vi "Version_2.0_Single_Column_Code.vi"() -> ()   [LabVIEW 2020] (continued)
                              frame #4 {
                                n4126 = while {
                                stop <- w4536 stop-if-true
                                n4127 = local read "Stopper that ends \nthe main loops"() -> (w4537:bool)
                                n4128 = local read "VISA Refnum in\nfor Pump"() -> (w4538:refnum<visa-resource-name>)
                                n4129 = case shown="True" w4537 {
                                frame False {
                                }
                                frame True {
                                n4130 = local read "VISA Refnum in\nfor Pump"() -> (w4539:refnum<visa-resource-name>)
                                n4131 = call "HardStopCurrentProcess (SubVI).vi"("VISA Refnum in"=w4539) -> ()  [unwired: 11 in]
                                }
                                }
                                n4132 = call "ProcessCompletionWaiterWithOutPut (SubVI).vi"("VISA Refnum in"=w4538) -> ("Boolean"=w4536:bool)  [unwired: 10 in]
                                }
                              }
                              frame #5 {
                                n4133 = local read "Buffer-B Dispense\nFlow Rate for Elution \ntubing pre-wash"() -> (w4543:dbl)
                                n4134 = local read "Buffer-B Pumping\nResolution"() -> (w4542:T2)
                                n4135 = local read "VISA Refnum in\nfor Pump"() -> (w4545:refnum<visa-resource-name>)
                                n4136 = local write "Pause Data Collection"(TRUE ("Pause Data Collection")) -> ()
                                n4137 = local read "Volume of Syringe"() -> (w4544:dbl)
                                n4138 = call "GoToAbsolutePosition(SubVI).vi"("Absolute Volume Position in Syringe (in ul)"=0.0 ("Volume to be Dispensed"), "Volume of Syringe"=w4544, "Resolution of Pumping"=w4542, "Flow Rate (ul/min)"=w4543, "VISA Refnum in"=w4545) -> ()  [unwired: 6 in, 1 out]
                              }
                              frame #6 {
                                n4139 = local read "VISA Refnum in\nfor Pump"() -> (w4549:refnum<visa-resource-name>)
                                n4140 = local read "Initial Plunger Position"() -> (w4548:dbl)
                                n4141 = local read "Volume of Syringe"() -> (w4546:dbl)
                                n4142 = local read "Buffer-B Pumping\nResolution"() -> (w4547:T2)
                                n4143 = while {
                                tunnel: w4548 -> [w4556]
                                tunnel: w4549 -> [w4555]
                                tunnel: w4547 -> [w4554]
                                tunnel: w4546 -> [w4553]
                                stop <- w4551 stop-if-true
                                n4144 = stacked-sequence {
                                tunnel: w4556 -> [w4563 _]
                                tunnel: w4555 -> [w4562 w4583]
                                tunnel: w4554 -> [w4561 _]
                                tunnel: w4553 -> [w4560 _]
                                tunnel: [_ w4581] -> w4551
                                frame #0 {
                                n4145 = call "AbsolutePlungerPosition (SubVI).vi"("VISA Refnum in"=w4562) -> ("Plunger Position"=w4559:i32)  [unwired: 10 in]
                                n4146 = case shown="\"Standard Pumping\", Default" w4561 {
                                tunnel: w4563 -> [w4568 w4577]
                                tunnel: w4559 -> [w4569 w4576]
                                tunnel: [w4567 w4574] -> w4558
                                tunnel: w4560 -> [w4566 w4575]
                                frame "Standard Pumping", Default {
                                n4147 = Subtract(x=w4568, y=w4569) -> (x-y=w4565:dbl)
                                n4148 = Absolute Value(x=w4565) -> (abs(x)=w4564:dbl)
                                n4149 = Multiply(x=w4564, y=w4566) -> (x*y=w4571:dbl)
                                n4150 = Divide(x=w4571, y=3000.0) -> (x/y=w4567:dbl)
                                }
                                frame "High Resolution Pumping" {
                                n4151 = Subtract(x=w4577, y=w4576) -> (x-y=w4573:dbl)
                                n4152 = Absolute Value(x=w4573) -> (abs(x)=w4572:dbl)
                                n4153 = Multiply(x=w4572, y=w4575) -> (x*y=w4579:dbl)
                                n4154 = Divide(x=w4579, y=24000.0) -> (x/y=w4574:dbl)
                                }
                                }
                                n4155 = local write "Volume being Injected \nin this process"(w4558) -> ()
                                }
                                frame #1 {
                                n4156 = call "LSPOneStatus (SubVI).vi"("VISA Refnum in"=w4583) -> ("read buffer"=w4585:string)  [unwired: 10 in]
                                n4157 = call <vilib>:"Trim Whitespace.vi"("string"=w4585) -> ("trimmed string"=w4584:string)  [unwired: 1 in]
                                n4158 = local read "Stopper that ends \nthe main loops"() -> (w4580:bool)
                                n4159 = Equal?(x=w4584, y="/0`\u0003") -> (x = y?=w4582:bool)
                                n4160 = Or(x=w4582, y=w4580) -> (x .or. y?=w4581:bool)
                                }
                                }
                                n4161 = Wait (ms)(milliseconds to wait=u32 100) -> ()  [unwired: 1 out]
                                n4162 = local read "Stopper that ends \nthe main loops"() -> (w4550:bool)
                                n4163 = case shown="True" w4550 {
                                frame False {
                                }
                                frame True {
                                n4164 = local read "VISA Refnum in\nfor Pump"() -> (w4557:refnum<visa-resource-name>)
                                n4165 = call "HardStopCurrentProcess (SubVI).vi"("VISA Refnum in"=w4557) -> ()  [unwired: 11 in]
                                }
                                }
                                }
                              }
                              frame #7 {
                                # "Change the pump port to Buffer-A1 for equilibriation of column-1"
                                n4166 = local read "VISA Refnum in\nfor Pump"() -> (w4588:refnum<visa-resource-name>)
                                n4167 = local read "Port for \nA1-Equilibriation"() -> (w4587:string)
                                n4168 = local write "Pause Data Collection"(TRUE ("Pause Data Collection")) -> ()
                                n4169 = Wait (ms)(milliseconds to wait=u32 500) -> ()  [unwired: 1 out]
                                n4170 = call "PortChanger (SubVI).vi"("Port Number"=w4587, "VISA Refnum in"=w4588) -> ()  [unwired: 10 in]
                              }
                              frame #8 {
                                n4171 = local read "VISA Refnum in\nfor Pump"() -> (w4592:refnum<visa-resource-name>)
                                n4172 = local write "Volume being Injected \nin this process"(0.0 ("Volume being Injected \nin this process")) -> ()
                                n4173 = call "ProcessCompletionWaiter (SubVI).vi"("VISA Refnum in"=w4592) -> ()  [unwired: 11 in]
                                n4174 = local write "Start the Process"(FALSE ("Start the Process")) -> ()
                              }
                            }
                          }
                          frame #7 {
                            # "Clean the tubing with Buffer-A1"
                            n4175 = local read "N-A1"() -> (w4594:i32)
                            n4176 = for {
                              N: w4594 -> [_]
                              n4177 = stacked-sequence {
                                frame #0 {
                                n4178 = local read "VISA Refnum in\nfor Pump"() -> (w4597:refnum<visa-resource-name>)
                                n4179 = local read "Port for \nA1-Equilibriation"() -> (w4596:string)
                                n4180 = call "PortChanger (SubVI).vi"("Port Number"=w4596, "VISA Refnum in"=w4597) -> ()  [unwired: 10 in]
                                }
                                frame #1 {
                                n4181 = local read "VISA Refnum in\nfor Pump"() -> (w4598:refnum<visa-resource-name>)
                                n4182 = call "ProcessCompletionWaiter (SubVI).vi"("VISA Refnum in"=w4598) -> ()  [unwired: 11 in]
                                }
                                frame #2 {
                                n4183 = local read "VISA Refnum in\nfor Pump"() -> (w4603:refnum<visa-resource-name>)
                                n4184 = local read "Apparent Volume\nof Syringe"() -> (w4599:dbl)
                                n4185 = local read "Volume of Syringe"() -> (w4600:dbl)
                                n4186 = call "RPickUp(SubVI).vi"("Volume to be picked up"=w4599, "Volume of Syringe"=w4600, "Resolution of PickUP"=T2."Standard Pumping", "PickUp Flow Rate (ul/min)"=150.0, "VISA Refnum in"=w4603) -> ()  [unwired: 6 in, 1 out]
                                }
                                frame #3 {
                                n4187 = local read "Stopper that ends \nthe main loops"() -> (w4604:bool)
                                n4188 = local read "VISA Refnum in\nfor Pump"() -> (w4605:refnum<visa-resource-name>)
                                n4189 = case shown="True" w4604 {
                                frame False {
                                }
                                frame True {
                                n4190 = local read "VISA Refnum in\nfor Pump"() -> (w4606:refnum<visa-resource-name>)
                                n4191 = call "HardStopCurrentProcess (SubVI).vi"("VISA Refnum in"=w4606) -> ()  [unwired: 11 in]
                                }
                                }
                                n4192 = call "ProcessCompletionWaiter (SubVI).vi"("VISA Refnum in"=w4605) -> ()  [unwired: 11 in]
                                }
                                frame #4 {
                                n4193 = local read "VISA Refnum in\nfor Pump"() -> (w4608:refnum<visa-resource-name>)
                                n4194 = call "PortChanger (SubVI).vi"("Port Number"="1", "VISA Refnum in"=w4608) -> ()  [unwired: 10 in]
                                }
                                frame #5 {
                                n4195 = local read "Stopper that ends \nthe main loops"() -> (w4609:bool)
                                n4196 = local read "VISA Refnum in\nfor Pump"() -> (w4610:refnum<visa-resource-name>)
                                n4197 = case shown="True" w4609 {
                                frame False {
                                }
                                frame True {
                                n4198 = local read "VISA Refnum in\nfor Pump"() -> (w4611:refnum<visa-resource-name>)
                                n4199 = call "HardStopCurrentProcess (SubVI).vi"("VISA Refnum in"=w4611) -> ()  [unwired: 11 in]
                                }
                                }
                                n4200 = call "ProcessCompletionWaiter (SubVI).vi"("VISA Refnum in"=w4610) -> ()  [unwired: 11 in]
                                }
                                frame #6 {
                                n4201 = local read "VISA Refnum in\nfor Pump"() -> (w4616:refnum<visa-resource-name>)
                                n4202 = local read "Volume of Syringe"() -> (w4613:dbl)
                                n4203 = call "GoToAbsolutePosition(SubVI).vi"("Absolute Volume Position in Syringe (in ul)"=0.0 ("Volume to be picked up"), "Volume of Syringe"=w4613, "Resolution of Pumping"=T2."Standard Pumping" ("Resolution of PickUP"), "Flow Rate (ul/min)"=150.0 ("PickUp Flow Rate (ul/min)"), "VISA Refnum in"=w4616) -> ()  [unwired: 6 in, 1 out]
                                }
                                frame #7 {
                                n4204 = local read "Stopper that ends \nthe main loops"() -> (w4617:bool)
                                n4205 = local read "VISA Refnum in\nfor Pump"() -> (w4618:refnum<visa-resource-name>)
                                n4206 = case shown="True" w4617 {
                                frame False {
                                }
                                frame True {
                                n4207 = local read "VISA Refnum in\nfor Pump"() -> (w4619:refnum<visa-resource-name>)
                                n4208 = call "HardStopCurrentProcess (SubVI).vi"("VISA Refnum in"=w4619) -> ()  [unwired: 11 in]
                                }
                                }
                                n4209 = call "ProcessCompletionWaiter (SubVI).vi"("VISA Refnum in"=w4618) -> ()  [unwired: 11 in]
                                }
                              }
                              n4210 = local write "Pause Data Collection"(TRUE ("Pause Data Collection")) -> ()
                            }
                          }
                          frame #8 {
                            # "Switch to Port-4"
                            # "Port-4 of pump is connected to Buffer-A1"
                            n4211 = local read "Port for \nA1-Equilibriation"() -> (w4620:string)
                            n4212 = local read "VISA Refnum in\nfor Pump"() -> (w4621:refnum<visa-resource-name>)
                            n4213 = call "PortChanger (SubVI).vi"("Port Number"=w4620, "VISA Refnum in"=w4621) -> ()  [unwired: 10 in]
                          }
                          frame #9 {
                            n4214 = local read "VISA Refnum in\nfor Pump"() -> (w4622:refnum<visa-resource-name>)
                            n4215 = call "ProcessCompletionWaiter (SubVI).vi"("VISA Refnum in"=w4622) -> ()  [unwired: 11 in]
                          }
                          frame #10 {
                            # "External vale is temporarily connected to teh waste outlet in this code"
                            n4216 = local write "Valve V3 Open"(FALSE ("Valve V3 Open")) -> ()
                            n4217 = local write "Valve V4 Open"(FALSE ("Valve V4 Open")) -> ()
                            n4218 = local write "Valve V1 Open"(TRUE ("Valve V1 Open")) -> ()
                            n4219 = local write "Valve V2 Open"(TRUE ("Valve V2 Open")) -> ()
                            n4220 = local write "External Valve \nOpen"(TRUE ("External Valve \nOpen")) -> ()
                            n4221 = local write "Valve V8 Open"(FALSE ("Valve V8 Open")) -> ()
                            n4222 = local write "Valve V6 Open"(FALSE ("Valve V6 Open")) -> ()
                            n4223 = local write "Valve V5 Open"(FALSE ("Valve V5 Open")) -> ()
                            n4224 = local write "Valve V7 Open"(FALSE ("Valve V7 Open")) -> ()
                          }
                          frame #11 {
                            n4225 = local read "Buffer-A1 Volume \nto be  Pumped \nfor Equilibration\nof Column-1"() -> (w4635:dbl)
                            n4226 = local read "Apparent Volume\nof Syringe"() -> (w4632:dbl)
                            n4227 = Quotient & Remainder(x=w4635, y=w4632) -> (x-y*floor(x/y)=w4633:dbl, floor(x/y)=w4634:dbl)
                            n4228 = for {
                              N: w4634 -> [_]
                              n4229 = stacked-sequence {
                                frame #0 {
                                n4230 = local read "Buffer-A1 PickUp \nFlow Rate (ul/min)\nfor Equilibration \nof Column-1"() -> (w4638:dbl)
                                n4231 = local read "Buffer-A1 Pumping\nResolution \nfor Equilibration \nof Column-1"() -> (w4637:T2)
                                n4232 = local read "VISA Refnum in\nfor Pump"() -> (w4640:refnum<visa-resource-name>)
                                n4233 = local read "Apparent Volume\nof Syringe"() -> (w4636:dbl)
                                n4234 = local read "Volume of Syringe"() -> (w4639:dbl)
                                n4235 = call "RPickUp(SubVI).vi"("Volume to be picked up"=w4636, "Volume of Syringe"=w4639, "Resolution of PickUP"=w4637, "PickUp Flow Rate (ul/min)"=w4638, "VISA Refnum in"=w4640) -> ()  [unwired: 6 in, 1 out]
                                }
                                frame #1 {
                                n4236 = while {
                                stop <- w4641 stop-if-true
                                n4237 = local read "Stopper that ends \nthe main loops"() -> (w4642:bool)
                                n4238 = local read "VISA Refnum in\nfor Pump"() -> (w4643:refnum<visa-resource-name>)
                                n4239 = case shown="True" w4642 {
                                frame False {
                                }
                                frame True {
                                n4240 = local read "VISA Refnum in\nfor Pump"() -> (w4644:refnum<visa-resource-name>)
                                n4241 = call "HardStopCurrentProcess (SubVI).vi"("VISA Refnum in"=w4644) -> ()  [unwired: 11 in]
                                }
                                }
                                n4242 = call "ProcessCompletionWaiterWithOutPut (SubVI).vi"("VISA Refnum in"=w4643) -> ("Boolean"=w4641:bool)  [unwired: 10 in]
                                }
                                }
                                frame #2 {
                                # "Reads the initial Plunger Position for computing the volume dispensed"
                                n4243 = local read "VISA Refnum in\nfor Pump"() -> (w4646:refnum<visa-resource-name>)
                                n4244 = call "AbsolutePlungerPosition (SubVI).vi"("VISA Refnum in"=w4646) -> ("Plunger Position"=w4645:i32)  [unwired: 10 in]
                                n4245 = local write "Initial Plunger Position"(w4645) -> ()
                                }
                                frame #3 {
                                # "Switch to Port-2"
                                # "Port-2 of the pump is conncted to column-1 of chip"
                                n4246 = local read "VISA Refnum in\nfor Pump"() -> (w4648:refnum<visa-resource-name>)
                                n4247 = call "PortChanger (SubVI).vi"("Port Number"="2", "VISA Refnum in"=w4648) -> ()  [unwired: 10 in]
                                }
                                frame #4 {
                                n4248 = while {
                                stop <- w4649 stop-if-true
                                n4249 = local read "Stopper that ends \nthe main loops"() -> (w4650:bool)
                                n4250 = local read "VISA Refnum in\nfor Pump"() -> (w4651:refnum<visa-resource-name>)
                                n4251 = case shown="True" w4650 {
                                frame False {
                                }
                                frame True {
                                n4252 = local read "VISA Refnum in\nfor Pump"() -> (w4652:refnum<visa-resource-name>)
                                n4253 = call "HardStopCurrentProcess (SubVI).vi"("VISA Refnum in"=w4652) -> ()  [unwired: 11 in]
                                }
                                }
                                n4254 = call "ProcessCompletionWaiterWithOutPut (SubVI).vi"("VISA Refnum in"=w4651) -> ("Boolean"=w4649:bool)  [unwired: 10 in]
                                }
                                }
                                frame #5 {
                                n4255 = local read "Buffer-A1 Dispense\nFlow Rate (ul/min) \nfor Equilibration\nof Column-1"() -> (w4656:dbl)
                                n4256 = local read "Buffer-A1 Pumping\nResolution \nfor Equilibration \nof Column-1"() -> (w4655:T2)
                                n4257 = local read "VISA Refnum in\nfor Pump"() -> (w4658:refnum<visa-resource-name>)
                                n4258 = local write "Pause Data Collection"(FALSE ("Pause Data Collection")) -> ()
                                n4259 = local read "Volume of Syringe"() -> (w4657:dbl)
                                n4260 = call "GoToAbsolutePosition(SubVI).vi"("Absolute Volume Position in Syringe (in ul)"=0.0, "Volume of Syringe"=w4657, "Resolution of Pumping"=w4655, "Flow Rate (ul/min)"=w4656, "VISA Refnum in"=w4658) -> ()  [unwired: 6 in, 1 out]
                                }
                                frame #6 {
                                n4261 = local read "Buffer-A1 Pumping\nResolution \nfor Equilibration \nof Column-1"() -> (w4660:T2)
                                n4262 = local read "VISA Refnum in\nfor Pump"() -> (w4662:refnum<visa-resource-name>)
                                n4263 = local read "Initial Plunger Position"() -> (w4661:dbl)
                                n4264 = local read "Volume of Syringe"() -> (w4659:dbl)
                                n4265 = while {
                                tunnel: w4661 -> [w4669]
                                tunnel: w4662 -> [w4668]
                                tunnel: w4660 -> [w4667]
                                tunnel: w4659 -> [w4666]
                                stop <- w4664 stop-if-true
                                n4266 = stacked-sequence {
                                tunnel: w4669 -> [w4676 _]
                                tunnel: w4668 -> [w4675 w4696]
                                tunnel: w4667 -> [w4674 _]
                                tunnel: w4666 -> [w4673 _]
                                tunnel: [_ w4694] -> w4664
                                frame #0 {
                                n4267 = call "AbsolutePlungerPosition (SubVI).vi"("VISA Refnum in"=w4675) -> ("Plunger Position"=w4672:i32)  [unwired: 10 in]
                                n4268 = case shown="\"Standard Pumping\", Default" w4674 {
                                tunnel: w4676 -> [w4681 w4690]
                                tunnel: w4672 -> [w4682 w4689]
                                tunnel: [w4680 w4687] -> w4671
                                tunnel: w4673 -> [w4679 w4688]
                                frame "Standard Pumping", Default {
                                n4269 = Subtract(x=w4681, y=w4682) -> (x-y=w4678:dbl)
                                n4270 = Absolute Value(x=w4678) -> (abs(x)=w4677:dbl)
                                n4271 = Multiply(x=w4677, y=w4679) -> (x*y=w4684:dbl)
                                n4272 = Divide(x=w4684, y=3000.0) -> (x/y=w4680:dbl)
                                }
                                frame "High Resolution Pumping" {
                                n4273 = Subtract(x=w4690, y=w4689) -> (x-y=w4686:dbl)
                                n4274 = Absolute Value(x=w4686) -> (abs(x)=w4685:dbl)
                                n4275 = Multiply(x=w4685, y=w4688) -> (x*y=w4692:dbl)
                                n4276 = Divide(x=w4692, y=24000.0) -> (x/y=w4687:dbl)
                                }
                                }
                                n4277 = local write "Volume being Injected \nin this process"(w4671) -> ()
                                }
                                frame #1 {
                                n4278 = call "LSPOneStatus (SubVI).vi"("VISA Refnum in"=w4696) -> ("read buffer"=w4698:string)  [unwired: 10 in]
                                n4279 = call <vilib>:"Trim Whitespace.vi"("string"=w4698) -> ("trimmed string"=w4697:string)  [unwired: 1 in]
                                n4280 = local read "Stopper that ends \nthe main loops"() -> (w4693:bool)
                                n4281 = Equal?(x=w4697, y="/0`\u0003") -> (x = y?=w4695:bool)
                                n4282 = Or(x=w4695, y=w4693) -> (x .or. y?=w4694:bool)
                                }
                                }
                                n4283 = Wait (ms)(milliseconds to wait=u32 100) -> ()  [unwired: 1 out]
                                n4284 = local read "Stopper that ends \nthe main loops"() -> (w4663:bool)
                                n4285 = case shown="True" w4663 {
                                frame False {
                                }
                                frame True {
                                n4286 = local read "VISA Refnum in\nfor Pump"() -> (w4670:refnum<visa-resource-name>)
                                n4287 = call "HardStopCurrentProcess (SubVI).vi"("VISA Refnum in"=w4670) -> ()  [unwired: 11 in]
                                }
                                }
                                }
                                }
                                frame #7 {
                                # "Change the pump port back to Buffer-A1"
                                n4288 = local read "VISA Refnum in\nfor Pump"() -> (w4701:refnum<visa-resource-name>)
                                n4289 = local read "Port for \nA1-Equilibriation"() -> (w4700:string)
                                n4290 = local write "Pause Data Collection"(TRUE ("Pause Data Collection")) -> ()
                                n4291 = Wait (ms)(milliseconds to wait=u32 500) -> ()  [unwired: 1 out]
                                n4292 = call "PortChanger (SubVI).vi"("Port Number"=w4700, "VISA Refnum in"=w4701) -> ()  [unwired: 10 in]
                                }
                                frame #8 {
                                n4293 = local read "VISA Refnum in\nfor Pump"() -> (w4704:refnum<visa-resource-name>)
                                n4294 = local write "Volume being Injected \nin this process"(0.0 ("Volume being Injected \nin this process")) -> ()
                                n4295 = call "ProcessCompletionWaiter (SubVI).vi"("VISA Refnum in"=w4704) -> ()  [unwired: 11 in]
                                }
                              }
                            }
                            n4296 = local write "Reminder of the \nVolume to be \nPumped"(w4633) -> ()
                          }
                          frame #12 {
                            n4297 = stacked-sequence {
                              frame #0 {
                                n4298 = local read "Buffer-A1 PickUp \nFlow Rate (ul/min)\nfor Equilibration \nof Column-1"() -> (w4708:dbl)
                                n4299 = local read "Buffer-A1 Pumping\nResolution \nfor Equilibration \nof Column-1"() -> (w4707:T2)
                                n4300 = local read "VISA Refnum in\nfor Pump"() -> (w4710:refnum<visa-resource-name>)
                                n4301 = local read "Reminder of the \nVolume to be \nPumped"() -> (w4706:dbl)
                                n4302 = local read "Volume of Syringe"() -> (w4709:dbl)
                                n4303 = call "RPickUp(SubVI).vi"("Volume to be picked up"=w4706, "Volume of Syringe"=w4709, "Resolution of PickUP"=w4707, "PickUp Flow Rate (ul/min)"=w4708, "VISA Refnum in"=w4710) -> ()  [unwired: 6 in, 1 out]
                              }
                              frame #1 {
                                n4304 = while {
                                stop <- w4711 stop-if-true
                                n4305 = local read "Stopper that ends \nthe main loops"() -> (w4712:bool)
                                n4306 = local read "VISA Refnum in\nfor Pump"() -> (w4713:refnum<visa-resource-name>)
                                n4307 = case shown="True" w4712 {
                                frame False {
                                }
                                frame True {
                                n4308 = local read "VISA Refnum in\nfor Pump"() -> (w4714:refnum<visa-resource-name>)
                                n4309 = call "HardStopCurrentProcess (SubVI).vi"("VISA Refnum in"=w4714) -> ()  [unwired: 11 in]
                                }
                                }
                                n4310 = call "ProcessCompletionWaiterWithOutPut (SubVI).vi"("VISA Refnum in"=w4713) -> ("Boolean"=w4711:bool)  [unwired: 10 in]
                                }
                              }
                              frame #2 {
                                # "Reads the initial Plunger Position for computing the volume dispensed"
                                n4311 = local read "VISA Refnum in\nfor Pump"() -> (w4716:refnum<visa-resource-name>)
                                n4312 = call "AbsolutePlungerPosition (SubVI).vi"("VISA Refnum in"=w4716) -> ("Plunger Position"=w4715:i32)  [unwired: 10 in]
                                n4313 = local write "Initial Plunger Position"(w4715) -> ()
                              }
                              frame #3 {
                                # "Switch to Port-2"
                                # "Port-2 of the pump is conncted to column-1 of chip"
                                n4314 = local read "VISA Refnum in\nfor Pump"() -> (w4718:refnum<visa-resource-name>)
                                n4315 = call "PortChanger (SubVI).vi"("Port Number"="2", "VISA Refnum in"=w4718) -> ()  [unwired: 10 in]
                              }
                              frame #4 {
                                n4316 = while {
                                stop <- w4719 stop-if-true
                                n4317 = local read "Stopper that ends \nthe main loops"() -> (w4720:bool)
                                n4318 = local read "VISA Refnum in\nfor Pump"() -> (w4721:refnum<visa-resource-name>)
                                n4319 = case shown="True" w4720 {
                                frame False {
                                }
                                frame True {
                                n4320 = local read "VISA Refnum in\nfor Pump"() -> (w4722:refnum<visa-resource-name>)
                                n4321 = call "HardStopCurrentProcess (SubVI).vi"("VISA Refnum in"=w4722) -> ()  [unwired: 11 in]
                                }
                                }
                                n4322 = call "ProcessCompletionWaiterWithOutPut (SubVI).vi"("VISA Refnum in"=w4721) -> ("Boolean"=w4719:bool)  [unwired: 10 in]
                                }
                              }
                              frame #5 {
                                n4323 = local read "Buffer-A1 Pumping\nResolution \nfor Equilibration \nof Column-1"() -> (w4725:T2)
                                n4324 = local read "Buffer-A1 Dispense\nFlow Rate (ul/min) \nfor Equilibration\nof Column-1"() -> (w4726:dbl)
                                n4325 = local read "VISA Refnum in\nfor Pump"() -> (w4728:refnum<visa-resource-name>)
                                n4326 = local write "Pause Data Collection"(FALSE ("Pause Data Collection")) -> ()
                                n4327 = local read "Volume of Syringe"() -> (w4727:dbl)
                                n4328 = call "GoToAbsolutePosition(SubVI).vi"("Absolute Volume Position in Syringe (in ul)"=0.0 ("Volume to be Dispensed"), "Volume of Syringe"=w4727, "Resolution of Pumping"=w4725, "Flow Rate (ul/min)"=w4726, "VISA Refnum in"=w4728) -> ()  [unwired: 6 in, 1 out]
                              }
                              frame #6 {
                                n4329 = local read "Buffer-A1 Pumping\nResolution \nfor Equilibration \nof Column-1"() -> (w4730:T2)
                                n4330 = local read "VISA Refnum in\nfor Pump"() -> (w4732:refnum<visa-resource-name>)
                                n4331 = local read "Initial Plunger Position"() -> (w4731:dbl)
                                n4332 = local read "Volume of Syringe"() -> (w4729:dbl)
                                n4333 = while {
                                tunnel: w4731 -> [w4739]
                                tunnel: w4732 -> [w4738]
                                tunnel: w4730 -> [w4737]
                                tunnel: w4729 -> [w4736]
                                stop <- w4734 stop-if-true
                                n4334 = stacked-sequence {
                                tunnel: w4739 -> [w4746 _]
                                tunnel: w4738 -> [w4745 w4766]
                                tunnel: w4737 -> [w4744 _]
                                tunnel: w4736 -> [w4743 _]
                                tunnel: [_ w4764] -> w4734
                                frame #0 {
                                n4335 = call "AbsolutePlungerPosition (SubVI).vi"("VISA Refnum in"=w4745) -> ("Plunger Position"=w4742:i32)  [unwired: 10 in]
                                n4336 = case shown="\"Standard Pumping\", Default" w4744 {
                                tunnel: w4746 -> [w4751 w4760]
                                tunnel: w4742 -> [w4752 w4759]
                                tunnel: [w4750 w4757] -> w4741
                                tunnel: w4743 -> [w4749 w4758]
                                frame "Standard Pumping", Default {
                                n4337 = Subtract(x=w4751, y=w4752) -> (x-y=w4748:dbl)
                                n4338 = Absolute Value(x=w4748) -> (abs(x)=w4747:dbl)
                                n4339 = Multiply(x=w4747, y=w4749) -> (x*y=w4754:dbl)
                                n4340 = Divide(x=w4754, y=3000.0) -> (x/y=w4750:dbl)
                                }
                                frame "High Resolution Pumping" {
                                n4341 = Subtract(x=w4760, y=w4759) -> (x-y=w4756:dbl)
                                n4342 = Absolute Value(x=w4756) -> (abs(x)=w4755:dbl)
                                n4343 = Multiply(x=w4755, y=w4758) -> (x*y=w4762:dbl)
                                n4344 = Divide(x=w4762, y=24000.0) -> (x/y=w4757:dbl)
                                }
                                }
                                n4345 = local write "Volume being Injected \nin this process"(w4741) -> ()
                                }
                                frame #1 {
                                n4346 = call "LSPOneStatus (SubVI).vi"("VISA Refnum in"=w4766) -> ("read buffer"=w4768:string)  [unwired: 10 in]
                                n4347 = call <vilib>:"Trim Whitespace.vi"("string"=w4768) -> ("trimmed string"=w4767:string)  [unwired: 1 in]
                                n4348 = local read "Stopper that ends \nthe main loops"() -> (w4763:bool)
                                n4349 = Equal?(x=w4767, y="/0`\u0003") -> (x = y?=w4765:bool)
                                n4350 = Or(x=w4765, y=w4763) -> (x .or. y?=w4764:bool)
                                }
                                }
                                n4351 = Wait (ms)(milliseconds to wait=u32 100) -> ()  [unwired: 1 out]
                                n4352 = local read "Stopper that ends \nthe main loops"() -> (w4733:bool)
                                n4353 = case shown="True" w4733 {
                                frame False {
                                }
                                frame True {
                                n4354 = local read "VISA Refnum in\nfor Pump"() -> (w4740:refnum<visa-resource-name>)
                                n4355 = call "HardStopCurrentProcess (SubVI).vi"("VISA Refnum in"=w4740) -> ()  [unwired: 11 in]
                                }
                                }
                                }
                              }
                              frame #7 {
                                # "Change the pump port to Buffer-C1 for equilibriation of column-2"
                                n4356 = local read "VISA Refnum in\nfor Pump"() -> (w4771:refnum<visa-resource-name>)
                                n4357 = local read "Port for \nC1-Equilibriation"() -> (w4770:string)
                                n4358 = local write "Pause Data Collection"(TRUE ("Pause Data Collection")) -> ()
                                n4359 = Wait (ms)(milliseconds to wait=u32 500) -> ()  [unwired: 1 out]
                                n4360 = call "PortChanger (SubVI).vi"("Port Number"=w4770, "VISA Refnum in"=w4771) -> ()  [unwired: 10 in]
                              }
                              frame #8 {
                                n4361 = local read "VISA Refnum in\nfor Pump"() -> (w4775:refnum<visa-resource-name>)
                                n4362 = local write "Volume being Injected \nin this process"(0.0 ("Volume being Injected \nin this process")) -> ()
                                n4363 = call "ProcessCompletionWaiter (SubVI).vi"("VISA Refnum in"=w4775) -> ()  [unwired: 11 in]
                                n4364 = local write "Start the Process"(FALSE ("Start the Process")) -> ()
                              }
                            }
                          }
                          frame #13 {
                            # "Clean the tubing with Buffer-C1"
                            n4365 = local read "N-C1"() -> (w4778:i32)
                            n4366 = local write "Equilibriating \nColumn-1"(FALSE ("Equilibriating \nColumn-1")) -> ()
                            n4367 = for {
                              N: w4778 -> [_]
                              n4368 = stacked-sequence {
                                frame #0 {
                                n4369 = local read "Port for \nC1-Equilibriation"() -> (w4781:string)
                                n4370 = local read "VISA Refnum in\nfor Pump"() -> (w4782:refnum<visa-resource-name>)
                                n4371 = call "PortChanger (SubVI).vi"("Port Number"=w4781, "VISA Refnum in"=w4782) -> ()  [unwired: 10 in]
                                }
                                frame #1 {
                                n4372 = local read "VISA Refnum in\nfor Pump"() -> (w4783:refnum<visa-resource-name>)
                                n4373 = call "ProcessCompletionWaiter (SubVI).vi"("VISA Refnum in"=w4783) -> ()  [unwired: 11 in]
                                }
                                frame #2 {
                                n4374 = local read "VISA Refnum in\nfor Pump"() -> (w4788:refnum<visa-resource-name>)
                                n4375 = local read "Apparent Volume\nof Syringe"() -> (w4784:dbl)
                                n4376 = local read "Volume of Syringe"() -> (w4785:dbl)
                                n4377 = call "RPickUp(SubVI).vi"("Volume to be picked up"=w4784, "Volume of Syringe"=w4785, "Resolution of PickUP"=T2."Standard Pumping", "PickUp Flow Rate (ul/min)"=150.0, "VISA Refnum in"=w4788) -> ()  [unwired: 6 in, 1 out]
                                }
                                frame #3 {
                                n4378 = local read "Stopper that ends \nthe main loops"() -> (w4789:bool)
                                n4379 = local read "VISA Refnum in\nfor Pump"() -> (w4790:refnum<visa-resource-name>)
                                n4380 = case shown="True" w4789 {
                                frame False {
                                }
                                frame True {
                                n4381 = local read "VISA Refnum in\nfor Pump"() -> (w4791:refnum<visa-resource-name>)
                                n4382 = call "HardStopCurrentProcess (SubVI).vi"("VISA Refnum in"=w4791) -> ()  [unwired: 11 in]
                                }
                                }
                                n4383 = call "ProcessCompletionWaiter (SubVI).vi"("VISA Refnum in"=w4790) -> ()  [unwired: 11 in]
                                }
                                frame #4 {
                                n4384 = local read "VISA Refnum in\nfor Pump"() -> (w4793:refnum<visa-resource-name>)
                                n4385 = call "PortChanger (SubVI).vi"("Port Number"="1", "VISA Refnum in"=w4793) -> ()  [unwired: 10 in]
                                }
                                frame #5 {
                                n4386 = local read "Stopper that ends \nthe main loops"() -> (w4794:bool)
                                n4387 = local read "VISA Refnum in\nfor Pump"() -> (w4795:refnum<visa-resource-name>)
                                n4388 = case shown="True" w4794 {
                                frame False {
                                }
                                frame True {
                                n4389 = local read "VISA Refnum in\nfor Pump"() -> (w4796:refnum<visa-resource-name>)
                                n4390 = call "HardStopCurrentProcess (SubVI).vi"("VISA Refnum in"=w4796) -> ()  [unwired: 11 in]
                                }
                                }
                                n4391 = call "ProcessCompletionWaiter (SubVI).vi"("VISA Refnum in"=w4795) -> ()  [unwired: 11 in]
                                }
                                frame #6 {
                                n4392 = local read "VISA Refnum in\nfor Pump"() -> (w4801:refnum<visa-resource-name>)
                                n4393 = local read "Volume of Syringe"() -> (w4798:dbl)
                                n4394 = call "GoToAbsolutePosition(SubVI).vi"("Absolute Volume Position in Syringe (in ul)"=0.0 ("Volume to be picked up"), "Volume of Syringe"=w4798, "Resolution of Pumping"=T2."Standard Pumping" ("Resolution of PickUP"), "Flow Rate (ul/min)"=150.0 ("PickUp Flow Rate (ul/min)"), "VISA Refnum in"=w4801) -> ()  [unwired: 6 in, 1 out]
                                }
                                frame #7 {
                                n4395 = local read "Stopper that ends \nthe main loops"() -> (w4802:bool)
                                n4396 = local read "VISA Refnum in\nfor Pump"() -> (w4803:refnum<visa-resource-name>)
                                n4397 = case shown="True" w4802 {
                                frame False {
                                }
                                frame True {
                                n4398 = local read "VISA Refnum in\nfor Pump"() -> (w4804:refnum<visa-resource-name>)
                                n4399 = call "HardStopCurrentProcess (SubVI).vi"("VISA Refnum in"=w4804) -> ()  [unwired: 11 in]
                                }
                                }
                                n4400 = call "ProcessCompletionWaiter (SubVI).vi"("VISA Refnum in"=w4803) -> ()  [unwired: 11 in]
                                }
                              }
                            }
                            n4401 = local write "Pause Data Collection"(TRUE ("Pause Data Collection")) -> ()
                            n4402 = local write "Equilibriating \nColumn-2"(TRUE ("Equilibriating \nColumn-2")) -> ()
                          }
                          frame #14 {
                            n4403 = local read "Buffer-C1 Volume \nto be  Pumped \nfor Equilibration\nof Column-2"() -> (w4808:dbl)
                            n4404 = local read "Apparent Volume\nof Syringe"() -> (w4805:dbl)
                            n4405 = Quotient & Remainder(x=w4808, y=w4805) -> (x-y*floor(x/y)=w4806:dbl, floor(x/y)=w4807:dbl)
                            n4406 = for {
                              N: w4807 -> [_]
                              n4407 = stacked-sequence {
                                frame #0 {
                                n4408 = local read "VISA Refnum in\nfor Pump"() -> (w4810:refnum<visa-resource-name>)
                                n4409 = local read "Port for \nC1-Equilibriation"() -> (w4809:string)
                                n4410 = call "PortChanger (SubVI).vi"("Port Number"=w4809, "VISA Refnum in"=w4810) -> ()  [unwired: 10 in]
                                }
                                frame #1 {
                                n4411 = local read "VISA Refnum in\nfor Pump"() -> (w4811:refnum<visa-resource-name>)
                                n4412 = call "ProcessCompletionWaiter (SubVI).vi"("VISA Refnum in"=w4811) -> ()  [unwired: 11 in]
                                }
                                frame #2 {
                                n4413 = local read "Buffer-C1 PickUp \nFlow Rate (ul/min)\nfor Equilibration \nof Column-2"() -> (w4814:dbl)
                                n4414 = local read "Buffer-C1 Pumping\nResolution \nfor Equilibration \nof Column-2"() -> (w4813:T2)
                                n4415 = local read "VISA Refnum in\nfor Pump"() -> (w4816:refnum<visa-resource-name>)
                                n4416 = local read "Apparent Volume\nof Syringe"() -> (w4812:dbl)
                                n4417 = local read "Volume of Syringe"() -> (w4815:dbl)
                                n4418 = call "RPickUp(SubVI).vi"("Volume to be picked up"=w4812, "Volume of Syringe"=w4815, "Resolution of PickUP"=w4813, "PickUp Flow Rate (ul/min)"=w4814, "VISA Refnum in"=w4816) -> ()  [unwired: 6 in, 1 out]
                                }
                                frame #3 {
                                n4419 = while {
                                stop <- w4817 stop-if-true
                                n4420 = local read "Stopper that ends \nthe main loops"() -> (w4818:bool)
                                n4421 = local read "VISA Refnum in\nfor Pump"() -> (w4819:refnum<visa-resource-name>)
                                n4422 = case shown="True" w4818 {
                                frame False {
                                }
                                frame True {
                                n4423 = local read "VISA Refnum in\nfor Pump"() -> (w4820:refnum<visa-resource-name>)
                                n4424 = call "HardStopCurrentProcess (SubVI).vi"("VISA Refnum in"=w4820) -> ()  [unwired: 11 in]
                                }
                                }
                                n4425 = call "ProcessCompletionWaiterWithOutPut (SubVI).vi"("VISA Refnum in"=w4819) -> ("Boolean"=w4817:bool)  [unwired: 10 in]
                                }
                                }
                                frame #4 {
                                # "Reads the initial Plunger Position for computing the volume dispensed"
                                n4426 = local read "VISA Refnum in\nfor Pump"() -> (w4822:refnum<visa-resource-name>)
                                n4427 = call "AbsolutePlungerPosition (SubVI).vi"("VISA Refnum in"=w4822) -> ("Plunger Position"=w4821:i32)  [unwired: 10 in]
                                n4428 = local write "Initial Plunger Position"(w4821) -> ()
                                }
                                frame #5 {
                                # "Switch to Port-10"
                                # "Port-10 of the pump is conncted to column-2 of chip"
                                n4429 = local read "VISA Refnum in\nfor Pump"() -> (w4824:refnum<visa-resource-name>)
                                n4430 = call "PortChanger (SubVI).vi"("Port Number"="10", "VISA Refnum in"=w4824) -> ()  [unwired: 10 in]
                                }
                                frame #6 {
                                n4431 = while {
                                stop <- w4825 stop-if-true
                                n4432 = local read "Stopper that ends \nthe main loops"() -> (w4826:bool)
                                n4433 = local read "VISA Refnum in\nfor Pump"() -> (w4827:refnum<visa-resource-name>)
                                n4434 = case shown="True" w4826 {
                                frame False {
                                }
                                frame True {
                                n4435 = local read "VISA Refnum in\nfor Pump"() -> (w4828:refnum<visa-resource-name>)
                                n4436 = call "HardStopCurrentProcess (SubVI).vi"("VISA Refnum in"=w4828) -> ()  [unwired: 11 in]
                                }
                                }
                                n4437 = call "ProcessCompletionWaiterWithOutPut (SubVI).vi"("VISA Refnum in"=w4827) -> ("Boolean"=w4825:bool)  [unwired: 10 in]
                                }
                                }
                                frame #7 {
                                # "Buffer-C pumped for column non-interference"
                                # "Keeps the AMF valve after column-1 open and valve after column-2 closed"
                                n4438 = local read "Buffer-C1 Dispense\nFlow Rate (ul/min) \nfor Equilibration\nof Column-2"() -> (w4841:dbl)
                                n4439 = local read "Buffer-C1 Pumping\nResolution \nfor Equilibration \nof Column-2"() -> (w4840:T2)
                                n4440 = local read "VISA Refnum in\nfor Pump"() -> (w4843:refnum<visa-resource-name>)
                                n4441 = local write "Pause Data Collection"(FALSE ("Pause Data Collection")) -> ()
                                n4442 = local read "Volume of Syringe"() -> (w4842:dbl)
                                n4443 = call "GoToAbsolutePosition(SubVI).vi"("Absolute Volume Position in Syringe (in ul)"=0.0, "Volume of Syringe"=w4842, "Resolution of Pumping"=w4840, "Flow Rate (ul/min)"=w4841, "VISA Refnum in"=w4843) -> ()  [unwired: 6 in, 1 out]
                                n4444 = local write "Valve V1 Open"(FALSE ("Valve V1 Open")) -> ()
                                n4445 = local write "Valve V2 Open"(TRUE ("Valve V2 Open")) -> ()
                                n4446 = local write "Valve V4 Open"(FALSE ("Valve V4 Open")) -> ()
                                n4447 = local write "Valve V3 Open"(TRUE ("Valve V3 Open")) -> ()
                                n4448 = local write "External Valve \nOpen"(TRUE ("External Valve \nOpen")) -> ()
                                n4449 = local write "Valve V5 Open"(FALSE ("Valve V5 Open")) -> ()
                                n4450 = local write "Valve V6 Open"(FALSE ("Valve V6 Open")) -> ()
                                n4451 = local write "Valve V7 Open"(FALSE ("Valve V7 Open")) -> ()
                                n4452 = local write "Valve V8 Open"(FALSE ("Valve V8 Open")) -> ()
                                }
                                frame #8 {
                                n4453 = local read "Buffer-C1 Pumping\nResolution \nfor Equilibration \nof Column-2"() -> (w4845:T2)
                                n4454 = local read "VISA Refnum in\nfor Pump"() -> (w4847:refnum<visa-resource-name>)
                                n4455 = local read "Initial Plunger Position"() -> (w4846:dbl)
                                n4456 = local read "Volume of Syringe"() -> (w4844:dbl)
                                n4457 = while {
                                tunnel: w4846 -> [w4854]
                                tunnel: w4847 -> [w4853]
                                tunnel: w4845 -> [w4852]
                                tunnel: w4844 -> [w4851]
                                stop <- w4849 stop-if-true
                                n4458 = stacked-sequence {
                                tunnel: w4854 -> [w4861 _]
                                tunnel: w4853 -> [w4860 w4885]
                                tunnel: w4852 -> [w4859 _]
                                tunnel: w4851 -> [w4858 _]
                                tunnel: [_ w4883] -> w4849
                                frame #0 {
                                n4459 = call "AbsolutePlungerPosition (SubVI).vi"("VISA Refnum in"=w4860) -> ("Plunger Position"=w4857:i32)  [unwired: 10 in]
                                n4460 = case shown="\"Standard Pumping\", Default" w4859 {
                                tunnel: w4861 -> [w4866 w4875]
                                tunnel: w4857 -> [w4867 w4874]
                                tunnel: [w4865 w4872] -> w4856
                                tunnel: w4858 -> [w4864 w4873]
                                frame "Standard Pumping", Default {
                                n4461 = Subtract(x=w4866, y=w4867) -> (x-y=w4863:dbl)
                                n4462 = Absolute Value(x=w4863) -> (abs(x)=w4862:dbl)
                                n4463 = Multiply(x=w4862, y=w4864) -> (x*y=w4869:dbl)
                                n4464 = Divide(x=w4869, y=3000.0) -> (x/y=w4865:dbl)
                                }
                                frame "High Resolution Pumping" {
                                n4465 = Subtract(x=w4875, y=w4874) -> (x-y=w4871:dbl)
                                n4466 = Absolute Value(x=w4871) -> (abs(x)=w4870:dbl)
                                n4467 = Multiply(x=w4870, y=w4873) -> (x*y=w4877:dbl)
                                n4468 = Divide(x=w4877, y=24000.0) -> (x/y=w4872:dbl)
                                }
                                }
                                n4469 = local write "Volume being Injected \nin this process"(w4856) -> ()
                                }
                                frame #1 {
                                n4470 = local read "Buffer-C Volume \nto be Pumped for\nColumn \nnon-interference"() -> (w4881:dbl)
                                n4471 = local read "Volume being Injected \nin this process"() -> (w4882:dbl)
                                n4472 = local read "Stopper that ends \nthe main loops"() -> (w4880:bool)
                                n4473 = call "LSPOneStatus (SubVI).vi"("VISA Refnum in"=w4885) -> ("read buffer"=w4887:string)  [unwired: 10 in]
                                n4474 = call <vilib>:"Trim Whitespace.vi"("string"=w4887) -> ("trimmed string"=w4886:string)  [unwired: 1 in]
                                n4475 = Equal?(x=w4886, y="/0`\u0003") -> (x = y?=w4884:bool)
                                n4476 = Greater Or Equal?(x=w4882, y=w4881) -> (x >= y?=w4879:bool)
                                n4477 = Or(x=w4880, y=w4879) -> (x .or. y?=w4878:bool)
                                n4478 = Or(x=w4884, y=w4878) -> (x .or. y?=w4883:bool)
                                }
                                }
                                n4479 = Wait (ms)(milliseconds to wait=u32 100) -> ()  [unwired: 1 out]
                                n4480 = local read "Stopper that ends \nthe main loops"() -> (w4848:bool)
                                n4481 = case shown="True" w4848 {
                                frame False {
                                }
                                frame True {
                                n4482 = local read "VISA Refnum in\nfor Pump"() -> (w4855:refnum<visa-resource-name>)
                                n4483 = call "HardStopCurrentProcess (SubVI).vi"("VISA Refnum in"=w4855) -> ()  [unwired: 11 in]
                                }
                                }
                                }
                                }
                                frame #9 {
                                n4484 = local write "Valve V3 Open"(TRUE ("Valve V3 Open")) -> ()
                                n4485 = local write "Valve V2 Open"(FALSE ("Valve V2 Open")) -> ()
                                n4486 = local write "Valve V4 Open"(TRUE ("Valve V1 Open")) -> ()
                                n4487 = local write "Valve V1 Open"(FALSE ("Valve V1 Open")) -> ()
                                n4488 = local write "External Valve \nOpen"(FALSE ("External Valve \nOpen")) -> ()
                                n4489 = local write "Valve V5 Open"(TRUE ("Valve V4 Open")) -> ()
                                n4490 = local write "Valve V8 Open"(FALSE ("Valve V8 Open")) -> ()
                                n4491 = local write "Valve V7 Open"(TRUE ("Valve V6 Open")) -> ()
                                n4492 = local write "Valve V6 Open"(FALSE ("Valve V6 Open")) -> ()
                                }
                                frame #10 {
                                n4493 = local read "Buffer-C1 Pumping\nResolution \nfor Equilibration \nof Column-2"() -> (w4899:T2)
                                n4494 = local read "VISA Refnum in\nfor Pump"() -> (w4901:refnum<visa-resource-name>)
                                n4495 = local read "Initial Plunger Position"() -> (w4900:dbl)
                                n4496 = local read "Volume of Syringe"() -> (w4898:dbl)
                                n4497 = while {
                                tunnel: w4900 -> [w4908]
                                tunnel: w4901 -> [w4907]
                                tunnel: w4899 -> [w4906]
                                tunnel: w4898 -> [w4905]
                                stop <- w4903 stop-if-true
                                n4498 = stacked-sequence {
                                tunnel: w4908 -> [w4915 _]
                                tunnel: w4907 -> [w4914 w4935]
                                tunnel: w4906 -> [w4913 _]
                                tunnel: w4905 -> [w4912 _]
                                tunnel: [_ w4933] -> w4903
                                frame #0 {
                                n4499 = call "AbsolutePlungerPosition (SubVI).vi"("VISA Refnum in"=w4914) -> ("Plunger Position"=w4911:i32)  [unwired: 10 in]
                                n4500 = case shown="\"Standard Pumping\", Default" w4913 {
                                tunnel: w4915 -> [w4920 w4929]
                                tunnel: w4911 -> [w4921 w4928]
                                tunnel: [w4919 w4926] -> w4910
                                tunnel: w4912 -> [w4918 w4927]
                                frame "Standard Pumping", Default {
                                n4501 = Subtract(x=w4920, y=w4921) -> (x-y=w4917:dbl)
                                n4502 = Absolute Value(x=w4917) -> (abs(x)=w4916:dbl)
                                n4503 = Multiply(x=w4916, y=w4918) -> (x*y=w4923:dbl)
                                n4504 = Divide(x=w4923, y=3000.0) -> (x/y=w4919:dbl)
                                }
                                frame "High Resolution Pumping" {
                                n4505 = Subtract(x=w4929, y=w4928) -> (x-y=w4925:dbl)
                                n4506 = Absolute Value(x=w4925) -> (abs(x)=w4924:dbl)
                                n4507 = Multiply(x=w4924, y=w4927) -> (x*y=w4931:dbl)
                                n4508 = Divide(x=w4931, y=24000.0) -> (x/y=w4926:dbl)
                                }
                                }
                                n4509 = local write "Volume being Injected \nin this process"(w4910) -> ()
                                }
                                frame #1 {
                                n4510 = local read "Stopper that ends \nthe main loops"() -> (w4932:bool)
                                n4511 = call "LSPOneStatus (SubVI).vi"("VISA Refnum in"=w4935) -> ("read buffer"=w4937:string)  [unwired: 10 in]
                                n4512 = call <vilib>:"Trim Whitespace.vi"("string"=w4937) -> ("trimmed string"=w4936:string)  [unwired: 1 in]
                                n4513 = Equal?(x=w4936, y="/0`\u0003") -> (x = y?=w4934:bool)
                                n4514 = Or(x=w4934, y=w4932) -> (x .or. y?=w4933:bool)
                                }
                                }
                                n4515 = Wait (ms)(milliseconds to wait=u32 100) -> ()  [unwired: 1 out]
                                n4516 = local read "Stopper that ends \nthe main loops"() -> (w4902:bool)
                                n4517 = case shown="True" w4902 {
                                frame False {
                                }
                                frame True {
                                n4518 = local read "VISA Refnum in\nfor Pump"() -> (w4909:refnum<visa-resource-name>)
                                n4519 = call "HardStopCurrentProcess (SubVI).vi"("VISA Refnum in"=w4909) -> ()  [unwired: 11 in]
                                }
                                }
                                }
                                }
                                frame #11 {
                                # "Change the pump port back to Buffer-C1"
                                n4520 = local read "VISA Refnum in\nfor Pump"() -> (w4940:refnum<visa-resource-name>)
                                n4521 = local read "Port for \nC1-Equilibriation"() -> (w4939:string)
                                n4522 = local write "Pause Data Collection"(TRUE ("Pause Data Collection")) -> ()
                                n4523 = Wait (ms)(milliseconds to wait=u32 500) -> ()  [unwired: 1 out]
                                n4524 = call "PortChanger (SubVI).vi"("Port Number"=w4939, "VISA Refnum in"=w4940) -> ()  [unwired: 10 in]
                                }
                                frame #12 {
                                n4525 = local read "VISA Refnum in\nfor Pump"() -> (w4943:refnum<visa-resource-name>)
                                n4526 = local write "Volume being Injected \nin this process"(0.0 ("Volume being Injected \nin this process")) -> ()
                                n4527 = call "ProcessCompletionWaiter (SubVI).vi"("VISA Refnum in"=w4943) -> ()  [unwired: 11 in]
                                }
                              }
                            }
                            n4528 = local write "Reminder of the \nVolume to be \nPumped"(w4806) -> ()
                          }
                          frame #15 {
                            n4529 = stacked-sequence {
                              frame #0 {
                                n4530 = local read "Buffer-C1 PickUp \nFlow Rate (ul/min)\nfor Equilibration \nof Column-2"() -> (w4947:dbl)
                                n4531 = local read "Buffer-C1 Pumping\nResolution \nfor Equilibration \nof Column-2"() -> (w4946:T2)
                                n4532 = local read "VISA Refnum in\nfor Pump"() -> (w4949:refnum<visa-resource-name>)
                                n4533 = local read "Reminder of the \nVolume to be \nPumped"() -> (w4945:dbl)
                                n4534 = local read "Volume of Syringe"() -> (w4948:dbl)
                                n4535 = call "RPickUp(SubVI).vi"("Volume to be picked up"=w4945, "Volume of Syringe"=w4948, "Resolution of PickUP"=w4946, "PickUp Flow Rate (ul/min)"=w4947, "VISA Refnum in"=w4949) -> ()  [unwired: 6 in, 1 out]
                              }
                              frame #1 {
                                n4536 = while {
                                stop <- w4950 stop-if-true
                                n4537 = local read "Stopper that ends \nthe main loops"() -> (w4951:bool)
                                n4538 = local read "VISA Refnum in\nfor Pump"() -> (w4952:refnum<visa-resource-name>)
                                n4539 = case shown="True" w4951 {
                                frame False {
                                }
                                frame True {
                                n4540 = local read "VISA Refnum in\nfor Pump"() -> (w4953:refnum<visa-resource-name>)
                                n4541 = call "HardStopCurrentProcess (SubVI).vi"("VISA Refnum in"=w4953) -> ()  [unwired: 11 in]
                                }
                                }
                                n4542 = call "ProcessCompletionWaiterWithOutPut (SubVI).vi"("VISA Refnum in"=w4952) -> ("Boolean"=w4950:bool)  [unwired: 10 in]
                                }
                              }
                              frame #2 {
                                # "Reads the initial Plunger Position for computing the volume dispensed"
                                n4543 = local read "VISA Refnum in\nfor Pump"() -> (w4955:refnum<visa-resource-name>)
                                n4544 = call "AbsolutePlungerPosition (SubVI).vi"("VISA Refnum in"=w4955) -> ("Plunger Position"=w4954:i32)  [unwired: 10 in]
                                n4545 = local write "Initial Plunger Position"(w4954) -> ()
                              }
                              frame #3 {
                                # "Switch to Port-10"
                                # "Port-10 of the pump is conncted to column-2 of chip"
                                n4546 = local read "VISA Refnum in\nfor Pump"() -> (w4957:refnum<visa-resource-name>)
                                n4547 = call "PortChanger (SubVI).vi"("Port Number"="10", "VISA Refnum in"=w4957) -> ()  [unwired: 10 in]
                              }
                              frame #4 {
                                n4548 = while {
                                stop <- w4958 stop-if-true
                                n4549 = local read "Stopper that ends \nthe main loops"() -> (w4959:bool)
                                n4550 = local read "VISA Refnum in\nfor Pump"() -> (w4960:refnum<visa-resource-name>)
                                n4551 = case shown="True" w4959 {
                                frame False {
                                }
                                frame True {
                                n4552 = local read "VISA Refnum in\nfor Pump"() -> (w4961:refnum<visa-resource-name>)
                                n4553 = call "HardStopCurrentProcess (SubVI).vi"("VISA Refnum in"=w4961) -> ()  [unwired: 11 in]
                                }
                                }
                                n4554 = call "ProcessCompletionWaiterWithOutPut (SubVI).vi"("VISA Refnum in"=w4960) -> ("Boolean"=w4958:bool)  [unwired: 10 in]
                                }
                              }
                              frame #5 {
                                # "Keeps the AMF valve after column-1 open and valve after column-2 closed"
                                n4555 = local read "Buffer-C1 Dispense\nFlow Rate (ul/min) \nfor Equilibration\nof Column-2"() -> (w4974:dbl)
                                n4556 = local read "Buffer-C1 Pumping\nResolution \nfor Equilibration \nof Column-2"() -> (w4973:T2)
                                n4557 = local read "VISA Refnum in\nfor Pump"() -> (w4976:refnum<visa-resource-name>)
                                n4558 = local write "Pause Data Collection"(FALSE ("Pause Data Collection")) -> ()
                                n4559 = local read "Volume of Syringe"() -> (w4975:dbl)
                                n4560 = call "GoToAbsolutePosition(SubVI).vi"("Absolute Volume Position in Syringe (in ul)"=0.0, "Volume of Syringe"=w4975, "Resolution of Pumping"=w4973, "Flow Rate (ul/min)"=w4974, "VISA Refnum in"=w4976) -> ()  [unwired: 6 in, 1 out]
                                n4561 = local write "Valve V1 Open"(FALSE ("Valve V1 Open")) -> ()
                                n4562 = local write "Valve V2 Open"(TRUE ("Valve V2 Open")) -> ()
                                n4563 = local write "Valve V3 Open"(TRUE ("Valve V3 Open")) -> ()
                                n4564 = local write "Valve V4 Open"(FALSE ("Affinity On")) -> ()
                                n4565 = local write "External Valve \nOpen"(TRUE ("External Valve \nOpen")) -> ()
                                n4566 = local write "Valve V8 Open"(FALSE ("Valve V8 Open")) -> ()
                                n4567 = local write "Valve V5 Open"(FALSE ("Valve V5 Open")) -> ()
                                n4568 = local write "Valve V6 Open"(FALSE ("Valve V6 Open")) -> ()
                                n4569 = local write "Valve V7 Open"(FALSE ("Valve V7 Open")) -> ()
                              }
                              frame #6 {
                                n4570 = local read "Buffer-C1 Pumping\nResolution \nfor Equilibration \nof Column-2"() -> (w4978:T2)
                                n4571 = local read "VISA Refnum in\nfor Pump"() -> (w4980:refnum<visa-resource-name>)
                                n4572 = local read "Initial Plunger Position"() -> (w4979:dbl)
                                n4573 = local read "Volume of Syringe"() -> (w4977:dbl)
                                n4574 = while {
                                tunnel: w4979 -> [w4987]
                                tunnel: w4980 -> [w4986]
                                tunnel: w4978 -> [w4985]
                                tunnel: w4977 -> [w4984]
                                stop <- w4982 stop-if-true
                                n4575 = stacked-sequence {
                                tunnel: w4987 -> [w4994 _]
                                tunnel: w4986 -> [w4993 w5018]
                                tunnel: w4985 -> [w4992 _]
                                tunnel: w4984 -> [w4991 _]
                                tunnel: [_ w5016] -> w4982
                                frame #0 {
                                n4576 = call "AbsolutePlungerPosition (SubVI).vi"("VISA Refnum in"=w4993) -> ("Plunger Position"=w4990:i32)  [unwired: 10 in]
                                n4577 = case shown="\"Standard Pumping\", Default" w4992 {
                                tunnel: w4994 -> [w4999 w5008]
                                tunnel: w4990 -> [w5000 w5007]
                                tunnel: [w4998 w5005] -> w4989
                                tunnel: w4991 -> [w4997 w5006]
                                frame "Standard Pumping", Default {
                                n4578 = Subtract(x=w4999, y=w5000) -> (x-y=w4996:dbl)
                                n4579 = Absolute Value(x=w4996) -> (abs(x)=w4995:dbl)
                                n4580 = Multiply(x=w4995, y=w4997) -> (x*y=w5002:dbl)
                                n4581 = Divide(x=w5002, y=3000.0) -> (x/y=w4998:dbl)
                                }
                                frame "High Resolution Pumping" {
                                n4582 = Subtract(x=w5008, y=w5007) -> (x-y=w5004:dbl)
                                n4583 = Absolute Value(x=w5004) -> (abs(x)=w5003:dbl)
                                n4584 = Multiply(x=w5003, y=w5006) -> (x*y=w5010:dbl)
                                n4585 = Divide(x=w5010, y=24000.0) -> (x/y=w5005:dbl)
                                }
                                }
                                n4586 = local write "Volume being Injected \nin this process"(w4989) -> ()
                                }
                                frame #1 {
                                n4587 = local read "Buffer-C Volume \nto be Pumped for\nColumn \nnon-interference"() -> (w5014:dbl)
                                n4588 = local read "Volume being Injected \nin this process"() -> (w5015:dbl)
                                n4589 = local read "Stopper that ends \nthe main loops"() -> (w5013:bool)
                                n4590 = call "LSPOneStatus (SubVI).vi"("VISA Refnum in"=w5018) -> ("read buffer"=w5020:string)  [unwired: 10 in]
                                n4591 = call <vilib>:"Trim Whitespace.vi"("string"=w5020) -> ("trimmed string"=w5019:string)  [unwired: 1 in]
                                n4592 = Equal?(x=w5019, y="/0`\u0003") -> (x = y?=w5017:bool)
                                n4593 = Greater Or Equal?(x=w5015, y=w5014) -> (x >= y?=w5012:bool)
                                n4594 = Or(x=w5013, y=w5012) -> (x .or. y?=w5011:bool)
                                n4595 = Or(x=w5017, y=w5011) -> (x .or. y?=w5016:bool)
                                }
                                }
                                n4596 = Wait (ms)(milliseconds to wait=u32 100) -> ()  [unwired: 1 out]
                                n4597 = local read "Stopper that ends \nthe main loops"() -> (w4981:bool)
                                n4598 = case shown="True" w4981 {
                                frame False {
                                }
                                frame True {
                                n4599 = local read "VISA Refnum in\nfor Pump"() -> (w4988:refnum<visa-resource-name>)
                                n4600 = call "HardStopCurrentProcess (SubVI).vi"("VISA Refnum in"=w4988) -> ()  [unwired: 11 in]
                                }
                                }
                                }
                              }
                              frame #7 {
                                n4601 = local write "Valve V4 Open"(TRUE ("Valve V4 Open")) -> ()
                                n4602 = local write "Valve V1 Open"(FALSE ("Valve V1 Open")) -> ()
                                n4603 = local write "Valve V2 Open"(FALSE ("Valve V2 Open")) -> ()
                                n4604 = local write "Valve V3 Open"(TRUE ("Valve V3 Open")) -> ()
                                n4605 = local write "External Valve \nOpen"(FALSE ("External Valve \nOpen")) -> ()
                                n4606 = local write "Valve V8 Open"(FALSE ("Valve V8 Open")) -> ()
                                n4607 = local write "Valve V7 Open"(TRUE ("Valve V7 Open")) -> ()
                                n4608 = local write "Valve V5 Open"(TRUE ("Valve V5 Open")) -> ()
                                n4609 = local write "Valve V6 Open"(TRUE ("Valve V6 Open")) -> ()
                              }
                              frame #8 {
                                n4610 = local read "Buffer-C1 Pumping\nResolution \nfor Equilibration \nof Column-2"() -> (w5032:T2)
                                n4611 = local read "VISA Refnum in\nfor Pump"() -> (w5034:refnum<visa-resource-name>)
                                n4612 = local read "Initial Plunger Position"() -> (w5033:dbl)
                                n4613 = local read "Volume of Syringe"() -> (w5031:dbl)
                                n4614 = while {
                                tunnel: w5033 -> [w5041]
                                tunnel: w5034 -> [w5040]
                                tunnel: w5032 -> [w5039]
                                tunnel: w5031 -> [w5038]
                                stop <- w5036 stop-if-true
                                n4615 = stacked-sequence {
                                tunnel: w5041 -> [w5048 _]
                                tunnel: w5040 -> [w5047 w5068]
                                tunnel: w5039 -> [w5046 _]
                                tunnel: w5038 -> [w5045 _]
                                tunnel: [_ w5066] -> w5036
                                frame #0 {
                                n4616 = call "AbsolutePlungerPosition (SubVI).vi"("VISA Refnum in"=w5047) -> ("Plunger Position"=w5044:i32)  [unwired: 10 in]
                                n4617 = case shown="\"Standard Pumping\", Default" w5046 {
                                tunnel: w5048 -> [w5053 w5062]
                                tunnel: w5044 -> [w5054 w5061]
                                tunnel: [w5052 w5059] -> w5043
                                tunnel: w5045 -> [w5051 w5060]
                                frame "Standard Pumping", Default {
                                n4618 = Subtract(x=w5053, y=w5054) -> (x-y=w5050:dbl)
                                n4619 = Absolute Value(x=w5050) -> (abs(x)=w5049:dbl)
                                n4620 = Multiply(x=w5049, y=w5051) -> (x*y=w5056:dbl)
                                n4621 = Divide(x=w5056, y=3000.0) -> (x/y=w5052:dbl)
                                }
                                frame "High Resolution Pumping" {
                                n4622 = Subtract(x=w5062, y=w5061) -> (x-y=w5058:dbl)
                                n4623 = Absolute Value(x=w5058) -> (abs(x)=w5057:dbl)
                                n4624 = Multiply(x=w5057, y=w5060) -> (x*y=w5064:dbl)
                                n4625 = Divide(x=w5064, y=24000.0) -> (x/y=w5059:dbl)
                                }
                                }
                                n4626 = local write "Volume being Injected \nin this process"(w5043) -> ()
                                }
                                frame #1 {
                                n4627 = local read "Stopper that ends \nthe main loops"() -> (w5065:bool)
                                n4628 = call "LSPOneStatus (SubVI).vi"("VISA Refnum in"=w5068) -> ("read buffer"=w5070:string)  [unwired: 10 in]
                                n4629 = call <vilib>:"Trim Whitespace.vi"("string"=w5070) -> ("trimmed string"=w5069:string)  [unwired: 1 in]
                                n4630 = Equal?(x=w5069, y="/0`\u0003") -> (x = y?=w5067:bool)
                                n4631 = Or(x=w5067, y=w5065) -> (x .or. y?=w5066:bool)
                                }
                                }
                                n4632 = Wait (ms)(milliseconds to wait=u32 100) -> ()  [unwired: 1 out]
                                n4633 = local read "Stopper that ends \nthe main loops"() -> (w5035:bool)
                                n4634 = case shown="True" w5035 {
                                frame False {
                                }
                                frame True {
                                n4635 = local read "VISA Refnum in\nfor Pump"() -> (w5042:refnum<visa-resource-name>)
                                n4636 = call "HardStopCurrentProcess (SubVI).vi"("VISA Refnum in"=w5042) -> ()  [unwired: 11 in]
                                }
                                }
                                }
                              }
                              frame #9 {
                                n4637 = local write "Pause Data Collection"(TRUE ("Pause Data Collection")) -> ()
                                n4638 = Wait (ms)(milliseconds to wait=u32 500) -> ()  [unwired: 1 out]
                              }
                              frame #10 {
                                n4639 = local write "Volume being Injected \nin this process"(0.0 ("Volume being Injected \nin this process")) -> ()
                                n4640 = local write "Start the Process"(FALSE ("Start the Process")) -> ()
                              }
                            }
                          }
                          frame #16 {
